vi "AttrSetMask.vi"(5 "LogSuspend":bool, 8 "error in":errorcluster, 10 "Value":u32, 11 "UdsHandleIn":T1={"LogPath"=path "", "LogEnabled"=FALSE, "isOpen"=FALSE, "LogContent"="", "Adapter"="CAN0", "MCanHandle"={"MCanAdapter"=refnum}, "TransmittId"=0, "ReceiveId"=0}) -> (0 "error out":errorcluster, 3 "UdsHandleOut":T1={"LogPath"=path "", "LogEnabled"=FALSE, "isOpen"=FALSE, "LogContent"="", "Adapter"="CAN0", "MCanHandle"={"MCanAdapter"=refnum}, "TransmittId"=0, "ReceiveId"=0})   [LabVIEW 2011, in "Konvolucio MUDS150628.lvlib"]
uses:
  <instrlib>/Konvolucio MUDS150628/Konvolucio MUDS150628.lvlib
  <instrlib>/Konvolucio MUDS150628/Types/UdsHandleType.ctl
  <instrlib>/Konvolucio MCAN120803/Types/MCanHandleType.ctl
  C:/Program Files/National Instruments/LabVIEW 2011/instr.lib/Konvolucio MCAN120803/Private/Konvolucio.MCAN120803.dll
  Konvolucio MCAN120803/Private/Konvolucio.MCAN120803.dll
  <instrlib>/Konvolucio MCAN120803/Konvolucio MCAN120803.lvlib
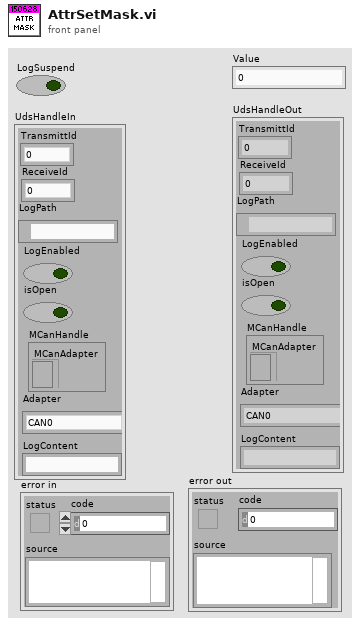
[diagram p1: front panel]
types:
  T1 = typedef "Konvolucio MUDS150628.lvlib/UdsHandleType.ctl" = cluster{"LogPath":path, "LogEnabled":bool, "isOpen":bool, "LogContent":string, "Adapter":string, "MCanHandle":T2, "TransmittId":u32, "ReceiveId":u32}
  T2 = typedef "Konvolucio MCAN120803.lvlib/MCanHandleType.ctl" = cluster{"MCanAdapter":refnum<k24>}
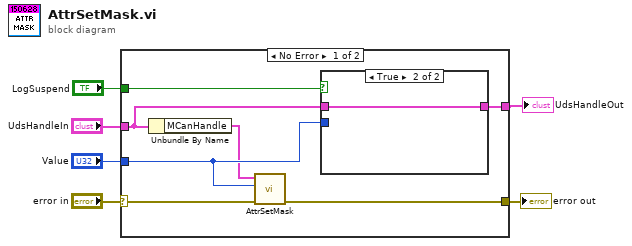
[diagram p0: block diagram]
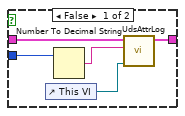
[diagram p2: hidden frame]
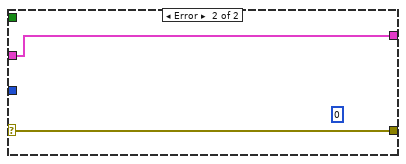
[diagram p3: hidden frame]
diagram:
  n1 = case shown="No Error" "error in" {
    selector: "error in" -> [w9 w21]
    tunnel: [w10 w21] -> w5
    tunnel: "UdsHandleIn" -> [w12 w20]
    tunnel: [w13 w20] -> w2
    tunnel: "LogSuspend" -> [w11 _]
    tunnel: "Value" -> [w8 _]
    frame No Error {
      n2 = Unbundle By Name(w12) -> ("MCanHandle"=w7:T2)
      n3 = call <instrlib>:"AttrSetMask.vi"("error in"=w9, "Value"=w8, "MCanHandleIn"=w7) -> ("error out"=w10:errorcluster)  [unwired: 6 in, 1 out]
      n4 = case shown="True" w11 {
        tunnel: w8 -> [w17 _]
        tunnel: [w16 w19] -> w13
        tunnel: w12 -> [w14 w19]
        frame False {
          n5 = control-ref of="This VI"() -> (w15:refnum<vi>)
          n6 = Number To Decimal String(number=w17) -> (decimal integer string=w18:string)  [unwired: 1 in]
          n7 = call <instrlib>:"UdsAttrLog.vi"("This VI"=w15, "Content"=w18, "UdsHandleIn"=w14) -> ("UdsHandleOut"=w16:T1)  [unwired: 8 in]
        }
        frame True {
        }
      }
    }
    frame Error {
      (unwired) u32 0 ("Attributes.RxErrorCounter")
    }
  }
  "error out" <- w5
  "UdsHandleOut" <- w2
